vi "send_json_http_post.vi"(8 "error in (no error)":errorcluster, 9 "timeout (10000)":i32 min=-1 step=1, 10 "URL":string, 11 "JSON":string) -> (0 "error out":errorcluster, 1 "body (server response)":string, 2 "headers":string, 3 "URL out":string)   [LabVIEW 2015]
uses:
  <vilib>/httpClient/POSTBuffer.vi
  <vilib>/httpClient/LabVIEWHTTPClient.lvlib
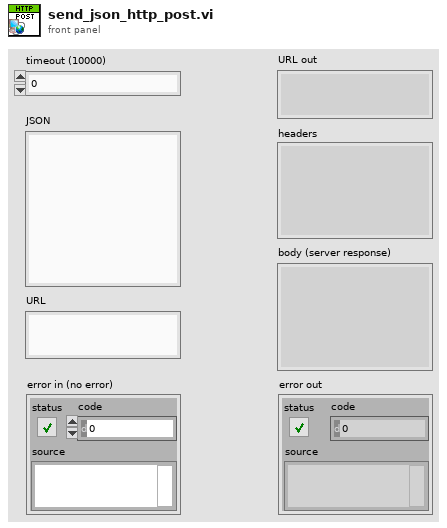
[diagram p1: front panel]
types:
  T1 = typedef "LabVIEWHTTPClient.lvlib/ClientHandle.ctl" = refnum<k1>
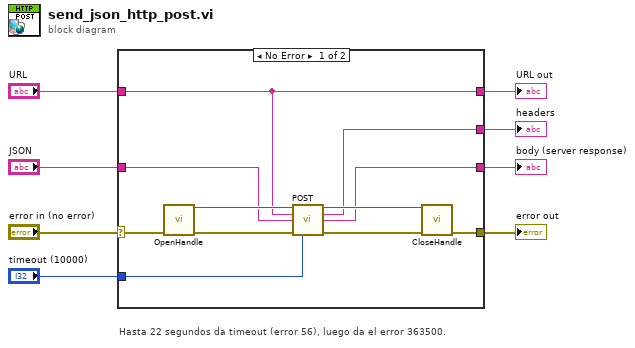
[diagram p0: block diagram]
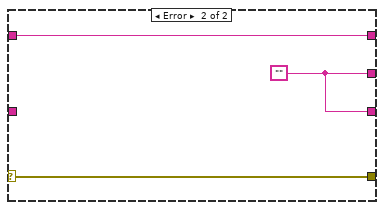
[diagram p2: hidden frame]
diagram:
  # "Hasta 22 segundos da timeout (error 56), luego da el error 363500."
  n1 = case shown="No Error" "error in (no error)" {
    selector: "error in (no error)" -> [w11 w22]
    tunnel: "timeout (10000)" -> [w19 _]
    tunnel: "URL" -> [w9 w20]
    tunnel: "JSON" -> [w14 _]
    tunnel: [w13 w21] -> w5
    tunnel: [w12 w22] -> w1
    tunnel: [w10 w21] -> w3
    tunnel: [w9 w20] -> w2
    frame No Error {
      n2 = call <vilib>:"OpenHandle.vi"("error in (no error)"=w11) -> ("client handle out"=w15:T1, "error out"=w16:errorcluster)  [unwired: 13 in]
      n3 = call-poly <vilib>:"POST.vi"("client handle"=w15, "url"=w9, "buffer"=w14, "error in (no error)"=w16, "timeout (10000)"=w19) -> ("client handle out"=w17:T1, "headers"=w10:string, "body"=w13:string, "error out"=w18:errorcluster)  [unwired: 7 in]
      n4 = call <vilib>:"CloseHandle.vi"("client handle"=w17, "error in (no error)"=w18) -> ("error out"=w12:errorcluster)  [unwired: 13 in]
    }
    frame Error {
      w21 = ""
    }
  }
  "error out" <- w1
  "body (server response)" <- w5
  "headers" <- w3
  "URL out" <- w2
